vi "Close.vi"(8 "error in (no error)":errorcluster, 11 "Data in":refnum<class "Omni_Bus.lvclass">) -> (0 "error out":errorcluster, 3 "Data out":refnum<class "Omni_Bus.lvclass">)   [LabVIEW 2021, in "Omni_Bus.lvclass"]
uses:
  Omni_Bus.lvclass
  Omni_Bus.lvclass/Omni_Bus.ctl
  Properties/Read Bus Access.vi
  Bus Access/Bus_Access.lvclass
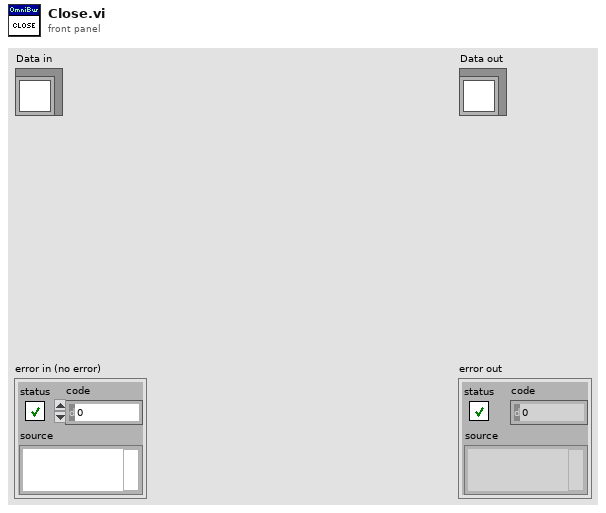
[diagram p1: front panel]
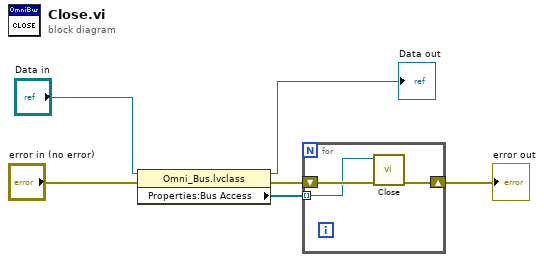
[diagram p0: block diagram]
diagram:
  n1 = property class="Omni_Bus.lvclass"(reference="Data in", error in="error in (no error)") -> (reference out=→"Data out":refnum<class "Omni_Bus.lvclass">, error out=w3:errorcluster, "Properties:Bus Access"=w4:refnum<class "Bus_Access.lvclass">[])
  n2 = for {
    tunnel: w4 -> [w8] mode=indexing
    shift-right: [w7] -> w1
    shift-left: w3 -> [w9]
    n3 = call-dynamic "Close.vi"("error in (no error)"=w9, "Data in"=w8) -> ("error out"=w7:errorcluster)  [unwired: 8 in, 1 out]
  }
  "error out" <- w1
